vi "PROJ_5-7.vi"() -> ()   [LabVIEW 2017]
panel:
  in  "Display History":bool
  in  "Size of Circle":i16
  in  "Send Button":bool
  in  "DAC 2":dbl
  in  "DAC1":dbl
  out "Y":dbl
  out "X":dbl
  in  "stop":bool
  out "2D Picture":picture
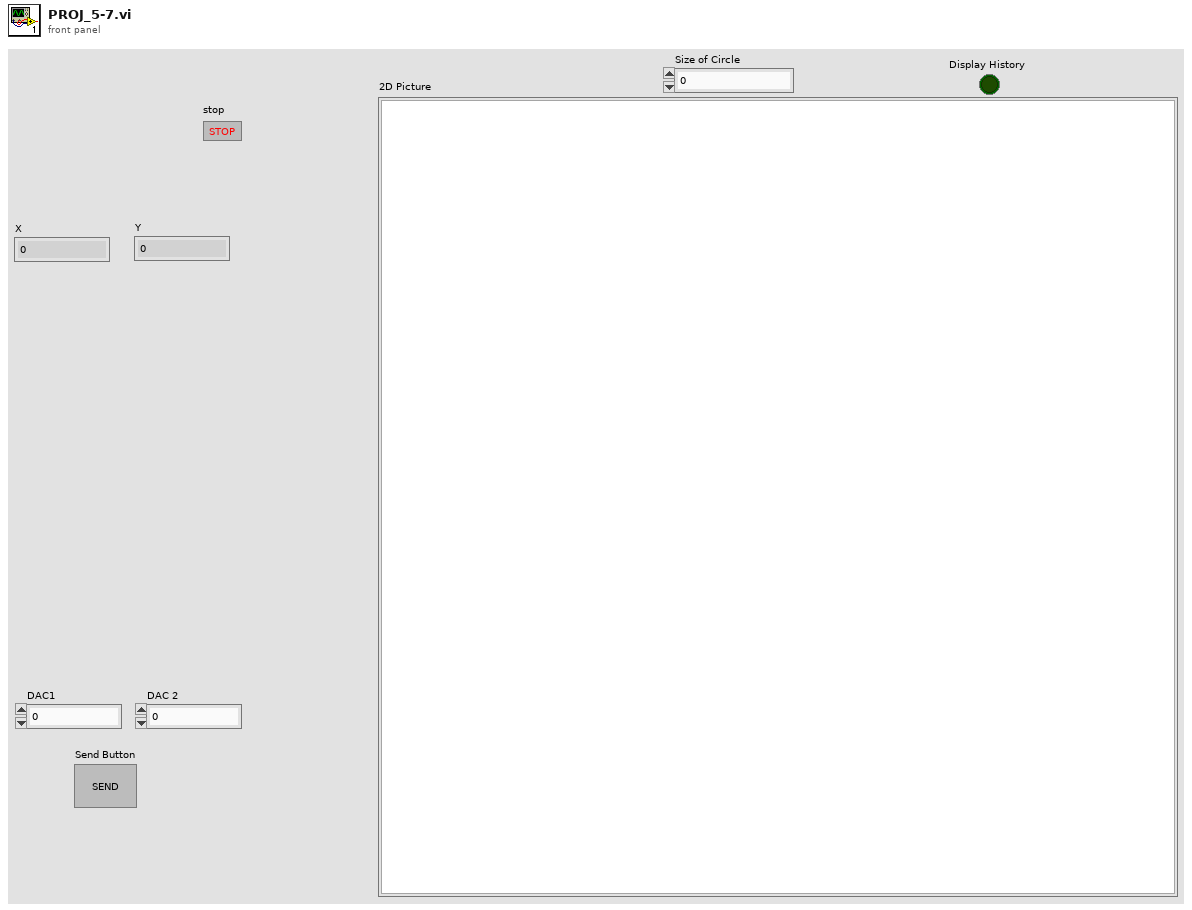
[diagram p1: front panel]
types:
  T1 = enum16{"Standard", "Buffered", "CRLF", "Immediate"}
  T2 = cluster{"Width":u16, "Style":enum32{"Solid", "Dash", "Dot", "DashDot", "DashDotDot"}}
  T3 = cluster{"default value 6":dbl, "default value 7":dbl}
  T4 = cluster{"default value 8":dbl, "default value 9":dbl}
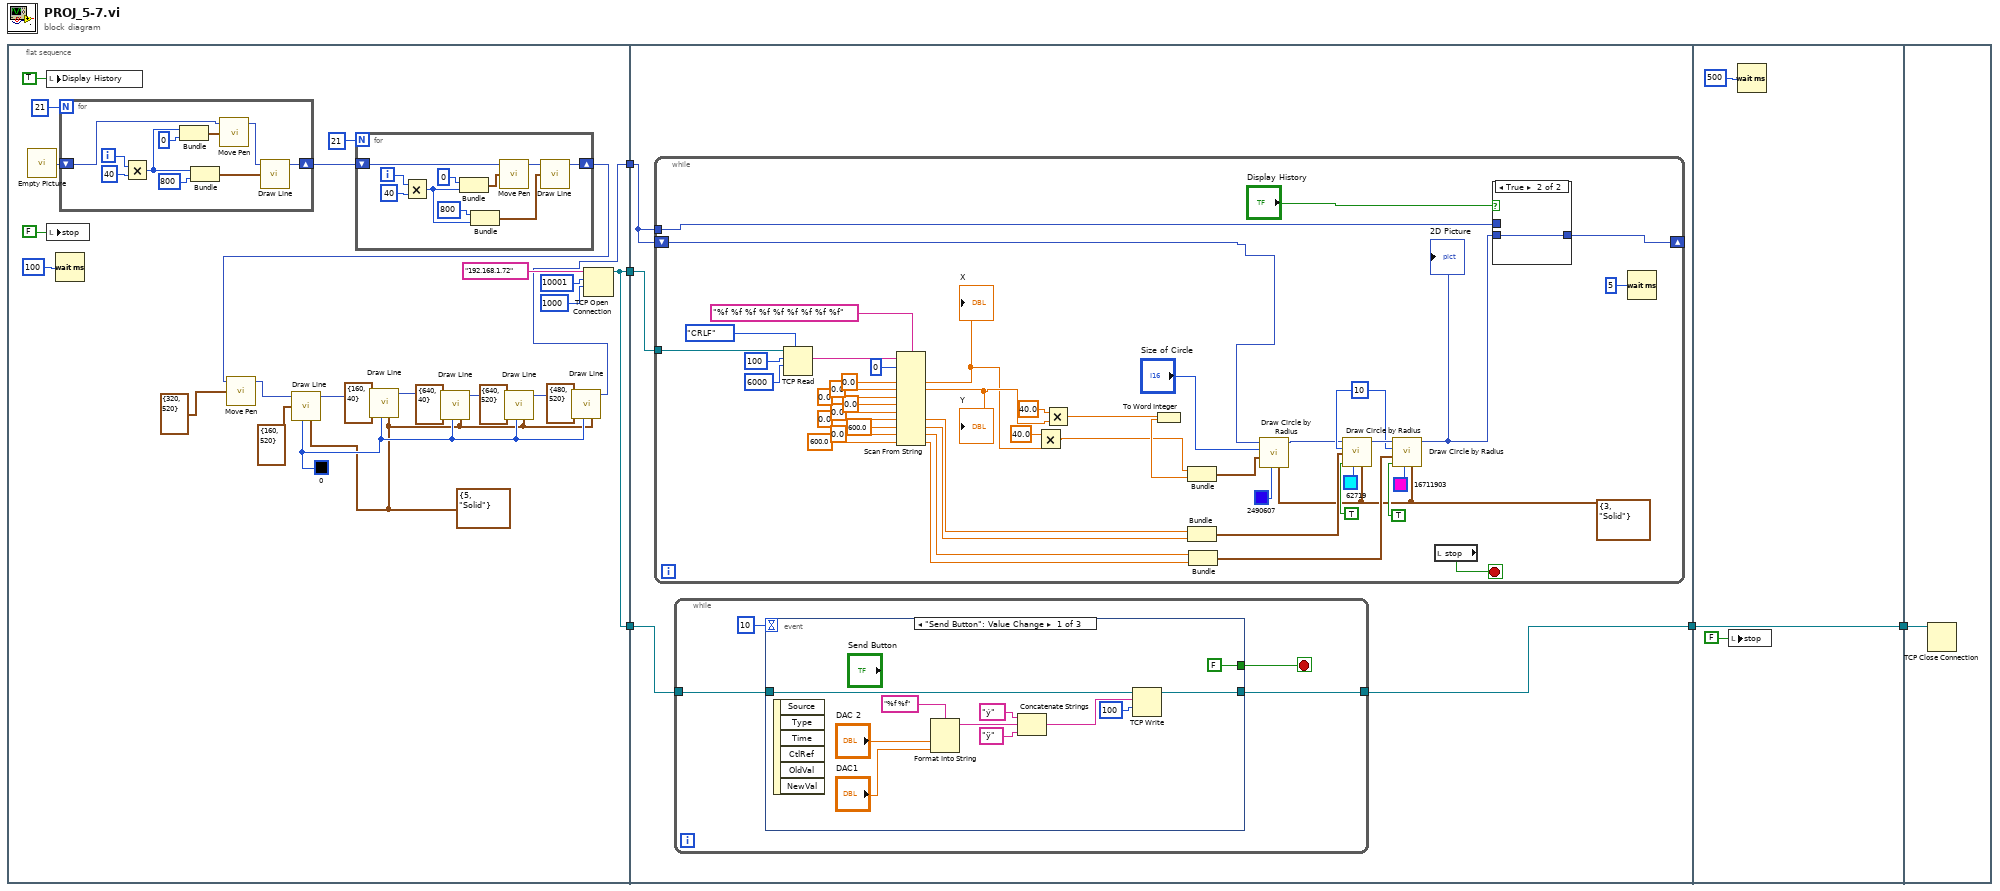
[diagram p0: block diagram]
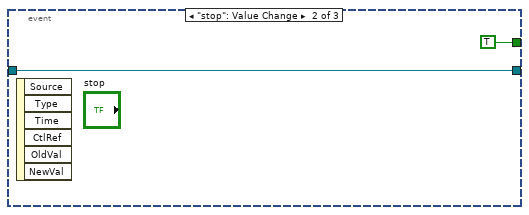
[diagram p3: hidden frame]
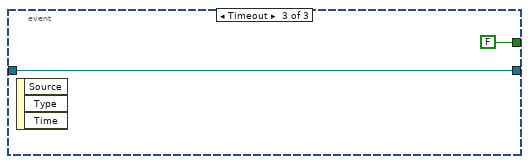
[diagram p4: hidden frame]
diagram:
  n1 = flat-sequence {
    tunnel: [w25] -> w5
    tunnel: [w25] -> w2
    tunnel: [w7] -> w1
    tunnel: w5 -> [w55]
    tunnel: [w54] -> w3
    tunnel: w2 -> [w53]
    tunnel: w1 -> [w52]
    tunnel: [w123] -> w4
    tunnel: w3 -> [w123]
    tunnel: w4 -> [w126]
    frame #0 {
      w13 = u32 0 ("color(black)")
      w6 = T2 {"Width"=5, "Style"=enum."Solid"} ("pen")
      n2 = call "Empty Picture"() -> ("empty picture"=w23:picture)
      n3 = local write "Display History"(TRUE ("Display History")) -> ()
      n4 = local write "stop"(FALSE ("stop")) -> ()
      n5 = Wait (ms)(milliseconds to wait=u32 100) -> ()  [unwired: 1 out]
      n6 = for {
        N: 21 -> [_]
        shift-right: [w49] -> w21
        shift-left: w23 -> [w50]
        i -> [w42]
        n7 = Multiply(x=w42, y=i16 40 ("x 2")) -> (x*y=w43:i32)
        n8 = Bundle(w43, 0) -> (w46:cluster{i32, i32})  [unwired: 1 in]
        n9 = Bundle(w43, 800) -> (w44:cluster{i32, i32})  [unwired: 1 in]
        n10 = call <vilib>:"Move Pen.vi"("new position"=w46, "picture"=w50) -> ("new picture"=w51:picture)  [unwired: 3 in]
        n11 = call <vilib>:"Draw Line.vi"("picture"=w51, "end point"=w44) -> ("new picture"=w49:picture)  [unwired: 7 in]
      }
      n12 = for {
        N: 21 -> [_]
        shift-right: [w39] -> w8
        shift-left: w21 -> [w40]
        i -> [w35]
        n13 = Multiply(x=w35, y=i16 40 ("x 2")) -> (x*y=w32:i32)
        n14 = Bundle(0, w32) -> (w37:cluster{i32, i32})  [unwired: 1 in]
        n15 = Bundle(800, w32) -> (w36:cluster{i32, i32})  [unwired: 1 in]
        n16 = call <vilib>:"Move Pen.vi"("new position"=w37, "picture"=w40) -> ("new picture"=w41:picture)  [unwired: 3 in]
        n17 = call <vilib>:"Draw Line.vi"("picture"=w41, "end point"=w36) -> ("new picture"=w39:picture)  [unwired: 7 in]
      }
      n18 = call <vilib>:"Move Pen.vi"("new position"=cluster{"x":i16, "y":i16} {"x"=320, "y"=520}, "picture"=w8) -> ("new picture"=w19:picture)  [unwired: 3 in]
      n19 = call <vilib>:"Draw Line.vi"("picture"=w19, "end point"=cluster{"x":i16, "y":i16} {"x"=160, "y"=520}, "color(black)"=w13, "pen"=w6) -> ("new picture"=w17:picture)  [unwired: 5 in]
      n20 = call <vilib>:"Draw Line.vi"("picture"=w17, "end point"=cluster{"x":i16, "y":i16} {"x"=160, "y"=40}, "color(black)"=w13, "pen"=w6) -> ("new picture"=w16:picture)  [unwired: 5 in]
      n21 = call <vilib>:"Draw Line.vi"("picture"=w16, "end point"=cluster{"x":i16, "y":i16} {"x"=640, "y"=40}, "color(black)"=w13, "pen"=w6) -> ("new picture"=w15:picture)  [unwired: 5 in]
      n22 = call <vilib>:"Draw Line.vi"("picture"=w15, "end point"=cluster{"x":i16, "y":i16} {"x"=640, "y"=520}, "color(black)"=w13, "pen"=w6) -> ("new picture"=w14:picture)  [unwired: 5 in]
      n23 = call <vilib>:"Draw Line.vi"("picture"=w14, "end point"=cluster{"x":i16, "y":i16} {"x"=480, "y"=520}, "color(black)"=w13, "pen"=w6) -> ("new picture"=w7:picture)  [unwired: 5 in]
      n24 = TCP Open Connection(address="192.168.1.72", remote port or service name=u16 10001, timeout ms (60000)=1000) -> (connection ID=w25:refnum<k5>)  [unwired: 2 in, 1 out]
    }
    frame #1 {
      n25 = while {
        tunnel: w53 -> [w101]
        shift-right: [w87] -> _
        shift-left: w52 -> [w56]
        tunnel: w52 -> [w86]
        stop <- w88 stop-if-true
        w67 = i16 10 ("radius")
        w58 = T2 {"Width"=3, "Style"=enum."Solid"} ("pen")
        n26 = TCP Read(connection ID=w101, bytes to read=100, 7:T1."CRLF" ("mode (standard)"), 9:6000 ("timeout ms (25000)")) -> (data out=w97:string)  [unwired: 1 in, 2 out]
        n27 = Scan From String(format string="%f %f %f %f %f %f %f %f %f", input string=w97, initial scan location=u32 0, default 1=0.0 ("default value 1"), default 2=0.0 ("default value 2"), default 3=0.0 ("default value 3"), default 4=0.0 ("default value 4"), default 5=0.0 ("default value 5"), default 6=0.0 ("default value 6"), default 7=600.0 ("default value 7"), default 8=0.0 ("default value 8"), default 9=600.0 ("default value 9")) -> (output 1=w81:dbl, output 2=w82:dbl, output 6=w73:dbl, output 7=w72:dbl, output 8=w65:dbl, output 9=w64:dbl)  [unwired: 4 in, 3 out]
        "Y" <- w82
        "X" <- w81
        n28 = Multiply(x=40.0, y=w81) -> (x*y=w83:dbl)
        n29 = Multiply(x=40.0, y=w82) -> (x*y=w84:dbl)
        n30 = To Word Integer(number=w84) -> ()  [unwired: 1 out]
        n31 = Bundle(w83, w84) -> (w61:cluster{dbl, dbl})  [unwired: 1 in]
        n32 = Bundle("default value 6"=w73, "default value 7"=w72) -> (w71:T3)  [unwired: 1 in]
        n33 = Bundle("default value 8"=w65, "default value 9"=w64) -> (w66:T4)  [unwired: 1 in]
        n34 = call <vilib>:"Draw Circle by Radius.vi"("pen"=w58, "color(black)"=u32 2490607, "pixel center"=w61, "radius"="Size of Circle", "picture"=w56) -> ("new picture"=w60:picture)  [unwired: 6 in]
        n35 = call <vilib>:"Draw Circle by Radius.vi"("pen"=w58, "color(black)"=u32 62719, "fill?(F)"=TRUE, "pixel center"=w71, "radius"=w67, "picture"=w60) -> ("new picture"=w69:picture)  [unwired: 5 in]
        n36 = call <vilib>:"Draw Circle by Radius.vi"("pen"=w58, "color(black)"=u32 16711903, "fill?(F)"=TRUE, "pixel center"=w66, "radius"=w67, "picture"=w69) -> ("new picture"=w70:picture)  [unwired: 5 in]
        "2D Picture" <- w70
        n37 = local read "stop"() -> (w88:bool)
        n38 = case shown="True" "Display History" {
          tunnel: w70 -> [_ w103]
          tunnel: [w102 w103] -> w87
          tunnel: w86 -> [w102 _]
          frame False {
          }
          frame True {
          }
        }
        n39 = Wait (ms)(milliseconds to wait=u32 5) -> ()  [unwired: 1 out]
      }
      n40 = while {
        tunnel: w55 -> [w106]
        tunnel: [w105] -> w54
        stop <- w104 stop-if-true
        n41 = event shown="[0] \"Send Button\": Value Change" {
          selector: _ -> [_ _ _]
          dyn-events: _ -> [_ _ _]
          timeout: 10 -> [_ _ _]
          tunnel: w106 -> [w110 w120 w122]
          tunnel: [w109 w120 w122] -> w105
          tunnel: [FALSE TRUE ("stop") FALSE] -> w104
          event "Send Button": Value Change {
            n42 = event-data() -> ()  [unwired: 1 in, 6 out]
            n43 = Format Into String(format string="%f %f", "DAC 2", "DAC1") -> (resulting string=w115:string)  [unwired: 2 in, 1 out]
            n44 = Concatenate Strings("ý" ("string"), w115, "ÿ" ("string")) -> (w112:string)
            n45 = TCP Write(connection ID=w110, data in=w112, 9:100 ("timeout ms (25000)")) -> (connection ID out=w109:refnum<k5>)  [unwired: 1 in, 2 out]
          }
          event "stop": Value Change {
            n46 = event-data() -> ()  [unwired: 1 in, 6 out]
          }
          event Timeout {
            n47 = event-data() -> ()  [unwired: 1 in, 3 out]
          }
        }
      }
    }
    frame #2 {
      n48 = local write "stop"(FALSE ("stop")) -> ()
      n49 = Wait (ms)(milliseconds to wait=u32 500) -> ()  [unwired: 1 out]
    }
    frame #3 {
      n50 = TCP Close Connection(connection ID=w126) -> ()  [unwired: 2 in, 2 out]
    }
  }
